vi "CopyClass.vi"(8 "error in (no error)":errorcluster, 9 "Actor Method VI Name":string, 10 "Subfolders":string, 11 "CS++Actor in":refnum<class "CS++Actor.lvclass">) -> (0 "error out":errorcluster, 1 "New Class Path":path, 2 "AddItemFromMemory":refnum<vi>, 3 "CS++Actor out":refnum<class "CS++Actor.lvclass">)   [LabVIEW 2014, in "CS++Actor.lvlib" / "CS++Actor.lvclass"]
doc: "Copies the template to the location of the new message class."
uses:
  CS++Actor.lvclass
  CS++Actor.lvclass/CS++Actor.ctl
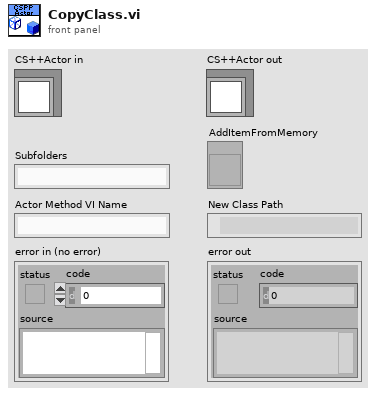
[diagram p1: front panel]
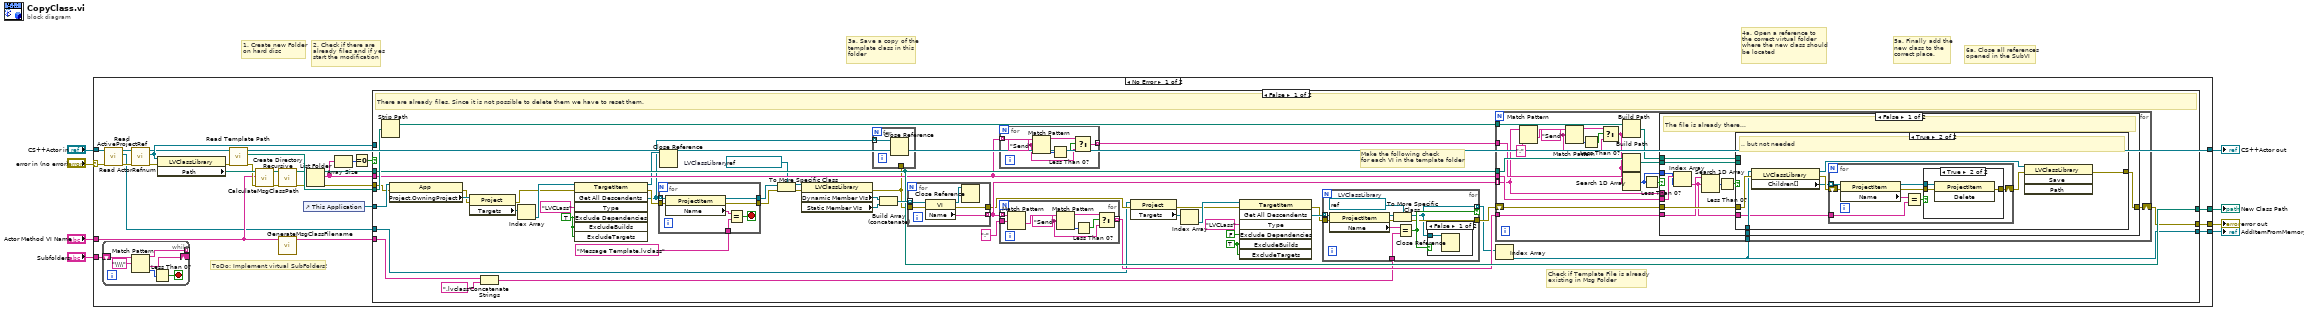
[diagram p0: block diagram]
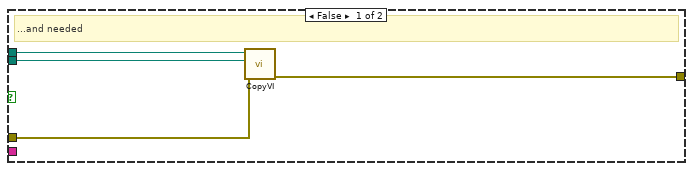
[diagram p3: hidden frame]
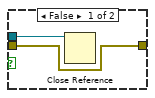
[diagram p4: hidden frame]
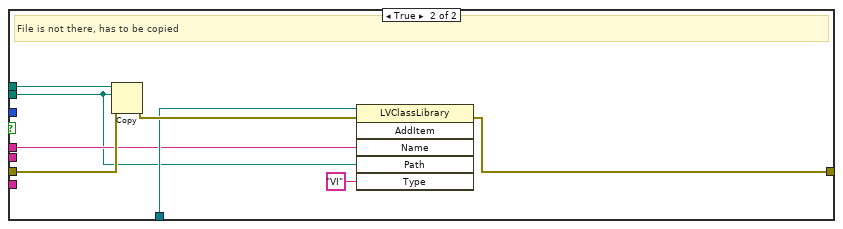
[diagram p5: hidden frame]
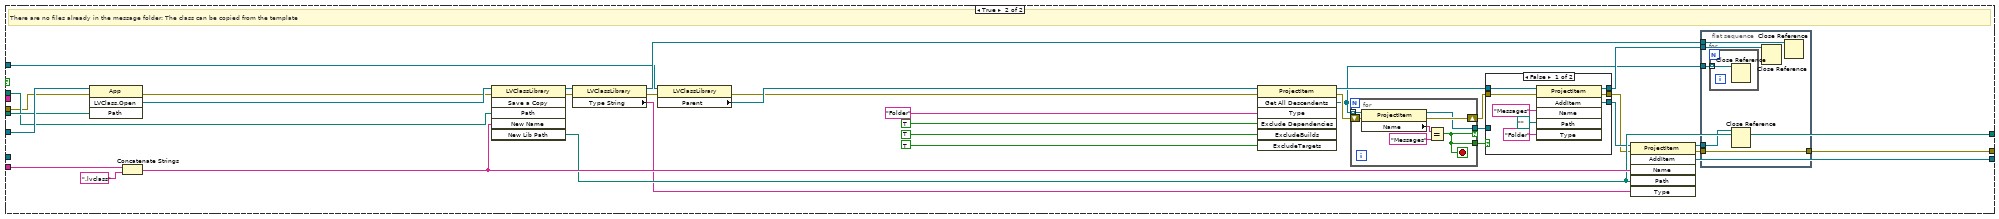
[diagram p6: hidden frame]
diagram:
  # "2. Check if there are\nalready files and if yes\nstart the modification"
  # "6a. Close all references\nopened in the SubVI"
  # "5a. Finally add the\nnew class to the\ncorrect place."
  # "4a. Open a reference to\nthe correct virtual folder\nwhere the new class should\nbe located"
  # "3a. Save a copy of the\ntemplate class in this \nfolder"
  # "1. Create new Folder\non hard disc"
  n1 = case shown="No Error" "error in (no error)" {
    selector: "error in (no error)" -> [w13 w253]
    tunnel: [w37 _] -> w8
    tunnel: "Actor Method VI Name" -> [w23 _]
    tunnel: [w29 w253] -> w6
    tunnel: [w36 _] -> w4
    tunnel: [w17 w252] -> w3
    tunnel: "CS++Actor in" -> [w10 w252]
    tunnel: "Subfolders" -> [w24 _]
    frame No Error {
      # "ToDo: Implement virtual SubFolders!"
      n2 = while {
        shift-right: [w249] -> _
        shift-left: w24 -> [w251]
        tunnel: [w248] -> _ mode=indexing
        stop <- w247 stop-if-true
        n3 = Match Pattern(string=w251, regular expression="\\\\") -> (before substring=w248:string, after substring=w249:string, offset past match=w246:i32)  [unwired: 1 in, 1 out]
        n4 = Less Than 0?(x=w246) -> (x < 0?=w247:bool)
      }
      n5 = call "Read ActiveProjectRef.vi"("error in (no error)"=w13, "CS++Actor in"=w10) -> ("error out"=w12:errorcluster, "ActiveProjectRef"=w9:refnum<vi>, "CS++Actor out"=w11:refnum<class "CS++Actor.lvclass">)  [unwired: 7 in]
      n6 = call "Read ActorRefnum.vi"("error in (no error)"=w12, "CS++Actor in"=w11) -> ("error out"=w35:errorcluster, "ActorRefnum"=w30:refnum<vi>, "CS++Actor out"=w26:refnum<class "CS++Actor.lvclass">)  [unwired: 7 in]
      n7 = property class="LVClassLibrary"(reference=w30, error in=w35) -> (error out=w28:errorcluster, "Path"=w34:path)  [unwired: 1 out]
      n8 = call "Read Template Path.vi"("error in (no error)"=w28, "CS++Actor in"=w26) -> ("error out"=w27:errorcluster, "Template Path"=w25:path, "CS++Actor out"=w17:refnum<class "CS++Actor.lvclass">)  [unwired: 7 in]
      n9 = call "CalculateMsgClassPath.vi"("error in (no error)"=w27, "Method VI Name"=w23, "Actor Class Path"=w34) -> ("error out"=w33:errorcluster, "Message Class Path"=w32:path)  [unwired: 7 in]
      n10 = call <vilib>:"Create Directory Recursive.vi"("error in (no error)"=w33, "directory"=w32) -> ("error out"=w20:errorcluster, "directory copy"=w21:path)  [unwired: 3 in, 1 out]
      n11 = call "GenerateMsgClassFilename.vi"("Target Method"=w23) -> ("Msg Class File Name"=w22:string)  [unwired: 10 in]
      n12 = control-ref of="This Application"() -> (w31:refnum<vi>)
      n13 = List Folder(path=w21, error in=w20) -> (path out=w18:path, filenames=w14:string[], error out=w16:errorcluster)  [unwired: 2 in, 1 out]
      n14 = Array Size(array=w14) -> (size(s)=w19:i32)
      n15 = Equal To 0?(x=w19) -> (x = 0?=w15:bool)
      n16 = case shown="False" w15 {
        tunnel: [w77 w217] -> w37
        tunnel: [w41 w212] -> w36
        tunnel: w31 -> [w71 w210]
        tunnel: w30 -> [_ w208]
        tunnel: [w76 w193] -> w29
        tunnel: w25 -> [w80 w190]
        tunnel: w22 -> [w78 w189]
        tunnel: w18 -> [w77 w188]
        tunnel: w16 -> [w70 w187]
        tunnel: w14 -> [w75 _]
        tunnel: w9 -> [w50 _]
        frame False {
          w40 = TRUE ("ExcludeDependencies")
          w63 = TRUE ("ExcludeDependencies")
          w56 = refnum<vi> refnum  # LVClassLibrary
          # "Check if Template File is already\nexisting in Msg Folder"
          # "Make the following check\nfor each VI in the template folder"
          # "There are already files. Since it is not possible to delete them we have to reset them."
          n17 = Strip Path(path=w80) -> (stripped path=w81:path)  [unwired: 1 out]
          n18 = property class="App"(reference=w71, error in=w70) -> (error out=w68:errorcluster, "Project.OwningProject"=w69:refnum<vi>)  [unwired: 1 out]
          n19 = property class="Project"(reference=w69, error in=w68) -> (error out=w65:errorcluster, "Targets"=w67:refnum<vi>[])  [unwired: 1 out]
          n20 = Concatenate Strings(w78, ".lvclass" ("regular expression")) -> (w43:string)
          n21 = Index Array(array=w67) -> (element=w66:refnum<vi>)  [unwired: 1 in]
          n22 = invoke class="TargetItem" method="Get All Descendents"(reference=w66, error in=w65, "Type"="LVCLass", "Exclude Dependencies"=w63, "ExcludeBuilds"=w63, "ExcludeTargets"=w63) -> (reference out=w55:refnum<vi>, error out=w61:errorcluster, "All Descendents"=w54:refnum<vi>[])  [unwired: 1 in, 4 out]
          n23 = for {
            tunnel: w54 -> [w103] mode=indexing
            tunnel: "Message Template.lvclass" ("Type") -> [w100]
            tunnel: [w99] -> w57
            tunnel: w61 -> [w98]
            tunnel: [w97] -> w59
            stop <- w101 stop-if-true
            n24 = property class="ProjectItem"(reference=w103, error in=w98) -> (reference out=w99:refnum<vi>, error out=w97:errorcluster, "Name"=w102:string)
            n25 = Equal?(x=w102, y=w100) -> (x = y?=w101:bool)
          }
          n26 = Close Reference(reference=w55) -> ()  [unwired: 1 in, 1 out]
          n27 = To More Specific Class(target class=w56, reference=w57, error in=w59) -> (specific class reference=w58:refnum<vi>, error out=w60:errorcluster)
          n28 = property class="LVClassLibrary"(reference=w58, error in=w60) -> (error out=w53:errorcluster, "Dynamic Member VIs"=w84:refnum<vi>[], "Static Member VIs"=w83:refnum<vi>[])  [unwired: 1 out]
          n29 = for {
            tunnel: w54 -> [w96] mode=indexing
            tunnel: w53 -> [_]
            n30 = Close Reference(reference=w96) -> ()  [unwired: 1 in, 1 out]
          }
          n31 = Build Array (concatenate)(w84, w83) -> (w82:refnum<vi>[])
          n32 = for {
            tunnel: w82 -> [w186] mode=indexing
            tunnel: [w182] -> w73 mode=indexing
            tunnel: w53 -> [w185]
            tunnel: [w184] -> w51
            n33 = property class="VI"(reference=w186, error in=w185) -> (reference out=w183:refnum<vi>, error out=w184:errorcluster, "Name"=w182:string)
            n34 = Close Reference(reference=w183) -> ()  [unwired: 1 in, 1 out]
          }
          n35 = for {
            tunnel: w75 -> [w112] mode=indexing
            tunnel: [w113] -> w74 mode=indexing
            w114 = "Send"
            n36 = Match Pattern(string=w112, regular expression=w114) -> (before substring=w115:string, offset past match=w117:i32)  [unwired: 1 in, 2 out]
            n37 = Less Than 0?(x=w117) -> (x < 0?=w116:bool)
            n38 = Select(t=w115, s=w116, f=w114) -> (s? t:f=w113:string)
          }
          n39 = for {
            tunnel: w73 -> [w106] mode=indexing
            tunnel: [w107] -> w72 mode=indexing
            tunnel: ":" ("regular expression") -> [w104]
            w111 = "Send"
            n40 = Match Pattern(string=w106, regular expression=w104) -> (after substring=w105:string)  [unwired: 1 in, 3 out]
            n41 = Match Pattern(string=w105, regular expression=w111) -> (before substring=w110:string, offset past match=w108:i32)  [unwired: 1 in, 2 out]
            n42 = Less Than 0?(x=w108) -> (x < 0?=w109:bool)
            n43 = Select(t=w110, s=w109, f=w111) -> (s? t:f=w107:string)
          }
          n44 = property class="Project"(reference=w50, error in=w51) -> (error out=w47:errorcluster, "Targets"=w52:refnum<vi>[])  [unwired: 1 out]
          n45 = Index Array(array=w52) -> (element=w48:refnum<vi>)  [unwired: 1 in]
          n46 = invoke class="TargetItem" method="Get All Descendents"(reference=w48, error in=w47, "Type"="LVCLass", "Exclude Dependencies"=FALSE ("ExcludeDependencies"), "ExcludeBuilds"=w40, "ExcludeTargets"=w40) -> (error out=w45:errorcluster, "All Descendents"=w46:refnum<vi>[])  [unwired: 1 in, 5 out]
          n47 = for {
            tunnel: w46 -> [w94] mode=indexing
            tunnel: w43 -> [w92]
            tunnel: [w86] -> w42 mode=indexing if=w90
            tunnel: w45 -> [w91]
            tunnel: [w88] -> w44
            w85 = refnum<vi> refnum  # LVClassLibrary
            n48 = property class="ProjectItem"(reference=w94, error in=w91) -> (reference out=w87:refnum<vi>, error out=w89:errorcluster, "Name"=w93:string)
            n49 = To More Specific Class(target class=w85, reference=w87, error in=w89) -> (specific class reference=w86:refnum<vi>, error out=w88:errorcluster)
            n50 = Equal?(x=w93, y=w92) -> (x = y?=w90:bool)
            n51 = case shown="False" w90 {
              tunnel: w86 -> [w95 _]
              frame False {
                n52 = Close Reference(reference=w95) -> ()  [unwired: 1 in, 1 out]
              }
              frame True {
              }
            }
          }
          n53 = Index Array(array=w42) -> (element=w41:refnum<vi>)  [unwired: 1 in]
          n54 = for {
            tunnel: w75 -> [w127]
            tunnel: w73 -> [w120] mode=indexing
            tunnel: w77 -> [w136]
            tunnel: w81 -> [w132]
            shift-right: [w131] -> w76
            shift-left: w44 -> [w133]
            tunnel: w41 -> [w130]
            tunnel: w72 -> [w129]
            tunnel: w74 -> [w126]
            w122 = "Send"
            n55 = Match Pattern(string=w120, regular expression=":") -> (after substring=w119:string)  [unwired: 1 in, 3 out]
            n56 = Match Pattern(string=w119, regular expression=w122) -> (before substring=w123:string, offset past match=w125:i32)  [unwired: 1 in, 2 out]
            n57 = Less Than 0?(x=w125) -> (x < 0?=w124:bool)
            n58 = Select(t=w123, s=w124, f=w122) -> (s? t:f=w121:string)
            n59 = Build Path(base path=w132, name or relative path=w121) -> (appended path=w134:path)
            n60 = Build Path(base path=w136, name or relative path=w121) -> (appended path=w135:path)
            n61 = Search 1D Array(1D array=w126, element=w121) -> (index of element=w128:i32)  [unwired: 1 in]
            n62 = Less Than 0?(x=w128) -> (x < 0?=w137:bool)
            n63 = case shown="False" w137 {
              tunnel: w135 -> [w148 w174]
              tunnel: w134 -> [w147 w181]
              tunnel: w133 -> [w146 w180]
              tunnel: [w145 w176] -> w131
              tunnel: w130 -> [w139 w177]
              tunnel: w120 -> [_ w175]
              tunnel: w129 -> [w143 _]
              tunnel: w127 -> [w141 _]
              tunnel: w128 -> [w140 _]
              frame False {
                # "The file is already there..."
                n64 = Index Array(array=w141, index=w140) -> (element=w138:string)
                n65 = Search 1D Array(1D array=w143, element=w138) -> (index of element=w144:i32)  [unwired: 1 in]
                n66 = Less Than 0?(x=w144) -> (x < 0?=w142:bool)
                n67 = case shown="True" w142 {
                  tunnel: w148 -> [w152 _]
                  tunnel: w147 -> [w151 _]
                  tunnel: w146 -> [w150 w160]
                  tunnel: [w149 w153] -> w145
                  tunnel: w139 -> [_ w159]
                  tunnel: w138 -> [_ w157]
                  frame False {
                    # "...and needed"
                    n68 = call "CopyVI.vi"("error in (no error)"=w150, "Empty File"=w152, "File to Copy"=w151) -> ("error out"=w149:errorcluster)  [unwired: 8 in]
                  }
                  frame True {
                    # ".. but not needed"
                    n69 = property class="LVClassLibrary"(reference=w159, error in=w160) -> (reference out=w156:refnum<vi>, error out=w158:errorcluster, "Children[]"=w155:refnum<vi>[])
                    n70 = for {
                      tunnel: w155 -> [w168] mode=indexing
                      shift-right: [w161] -> w154
                      shift-left: w158 -> [w167]
                      tunnel: w157 -> [w165]
                      n71 = property class="ProjectItem"(reference=w168, error in=w167) -> (reference out=w163:refnum<vi>, error out=w162:errorcluster, "Name"=w166:string)
                      n72 = Equal?(x=w166, y=w165) -> (x = y?=w164:bool)
                      n73 = case shown="True" w164 {
                        tunnel: w163 -> [w170 w173]
                        tunnel: w162 -> [w169 w172]
                        tunnel: [w169 w171] -> w161
                        frame False {
                          n74 = Close Reference(reference=w170) -> ()  [unwired: 1 in, 1 out]
                        }
                        frame True {
                          n75 = invoke class="ProjectItem" method="Delete"(reference=w173, error in=w172) -> (error out=w171:errorcluster)  [unwired: 1 in, 2 out]
                        }
                      }
                    }
                    n76 = invoke class="LVClassLibrary" method="Save"(reference=w156, error in=w154) -> (error out=w153:errorcluster)  [unwired: 2 in, 3 out]
                  }
                }
              }
              frame True {
                # "File is not there, has to be copied"
                n77 = Copy(8:w180, 10:w174, 11:w181) -> (0:w178:errorcluster)  [unwired: 2 in, 2 out]
                n78 = invoke class="LVClassLibrary" method="AddItem"(reference=w177, error in=w178, "Name"=w175, "Path"=w174, "Type"="VI") -> (error out=w176:errorcluster)  [unwired: 1 in, 5 out]
              }
            }
          }
        }
        frame True {
          # "There are no files already in the message folder: The class can be copied from the template"
          n79 = invoke class="App" method="LVClass.Open"(reference=w210, error in=w187, "Path"=w190) -> (error out=w220:errorcluster, "LVClass.Open"=w221:refnum<vi>)  [unwired: 1 in, 2 out]
          n80 = Concatenate Strings(w189, ".lvclass" ("regular expression")) -> (w218:string)
          n81 = invoke class="LVClassLibrary" method="Save a Copy"(reference=w221, error in=w220, "Path"=w188, "New Name"=w218) -> (reference out=w215:refnum<vi>, error out=w213:errorcluster, "New Lib Path"=w217:path)  [unwired: 2 in, 3 out]
          n82 = property class="LVClassLibrary"(reference=w215, error in=w213) -> (reference out=w214:refnum<vi>, error out=w209:errorcluster, "Type String"=w216:string)
          n83 = property class="LVClassLibrary"(reference=w208, error in=w209) -> (error out=w204:errorcluster, "Parent"=w206:refnum<vi>)  [unwired: 1 out]
          n84 = invoke class="ProjectItem" method="Get All Descendents"(reference=w206, error in=w204, "Type"="Folder", "Exclude Dependencies"=TRUE ("ExcludeDependencies"), "ExcludeBuilds"=TRUE, "ExcludeTargets"=TRUE) -> (reference out=w205:refnum<vi>, error out=w199:errorcluster, "All Descendents"=w194:refnum<vi>[])  [unwired: 1 in, 4 out]
          n85 = for {
            tunnel: w194 -> [w245] mode=indexing
            shift-right: [w243] -> w197
            shift-left: w199 -> [w244]
            tunnel: [w240] -> w196 if=w239
            tunnel: [w239] -> w198
            stop <- w239 stop-if-true
            n86 = property class="ProjectItem"(reference=w245, error in=w244) -> (reference out=w240:refnum<vi>, error out=w243:errorcluster, "Name"=w242:string)
            n87 = Equal?(x=w242, y="Messages") -> (x = y?=w239:bool)
          }
          n88 = case shown="False" w198 {
            tunnel: [w233 w238] -> w211
            tunnel: [w231 w237] -> w207
            tunnel: w205 -> [w230 w236]
            tunnel: w197 -> [w229 w237]
            tunnel: w196 -> [_ w238]
            tunnel: [w228 w236] -> w195
            frame False {
              n89 = invoke class="ProjectItem" method="AddItem"(reference=w230, error in=w229, "Name"="Messages", "Path"=path "", "Type"="Folder") -> (reference out=w228:refnum<vi>, error out=w231:errorcluster, "AddItem"=w233:refnum<vi>)  [unwired: 1 in, 3 out]
            }
            frame True {
            }
          }
          n90 = invoke class="ProjectItem" method="AddItem"(reference=w211, error in=w207, "Name"=w218, "Path"=w217, "Type"=w216) -> (reference out=w191:refnum<vi>, error out=w192:errorcluster, "AddItem"=w212:refnum<vi>)  [unwired: 1 in, 3 out]
          n91 = flat-sequence {
            tunnel: w214 -> [w226]
            tunnel: w195 -> [w225]
            tunnel: w194 -> [w224]
            tunnel: [w223] -> w193
            tunnel: w192 -> [w223]
            tunnel: w191 -> [w222]
            frame #0 {
              n92 = for {
                tunnel: w224 -> [w227] mode=indexing
                n93 = Close Reference(reference=w227) -> ()  [unwired: 1 in, 1 out]
              }
              n94 = Close Reference(reference=w222) -> ()  [unwired: 1 in, 1 out]
              n95 = Close Reference(reference=w225) -> ()  [unwired: 1 in, 1 out]
              n96 = Close Reference(reference=w226) -> ()  [unwired: 1 in, 1 out]
            }
          }
        }
      }
    }
    frame Error {
    }
  }
  "error out" <- w6
  "New Class Path" <- w8
  "AddItemFromMemory" <- w4
  "CS++Actor out" <- w3
